vi "Suscribe To Audio Spectrum Notifier.vi"(8 "Error In":errorcluster, 11 "Display Manager In":refnum<class "Display Manager.lvclass">) -> (0 "Error Out":errorcluster, 3 "Display Manager Out":refnum<class "Display Manager.lvclass">)   [LabVIEW 2019, in "Display Manager.lvclass"]
uses:
  Display Manager.lvclass
  Accessors/Audio Spectrum Notifier/Set Audio Spectrum Notifier.vi
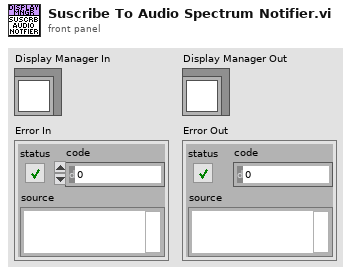
[diagram p1: front panel]
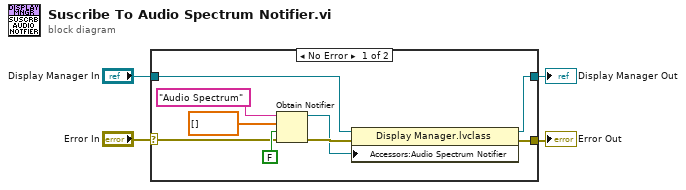
[diagram p0: block diagram]
diagram:
  n1 = case shown="No Error" "Error In" {
    selector: "Error In" -> [w7 w14]
    tunnel: [w13 w14] -> w4
    tunnel: [w12 w15] -> w3
    tunnel: "Display Manager In" -> [w9 w15]
    frame No Error {
      n2 = Obtain Notifier(name (unnamed)="Audio Spectrum", notification data type=dbl[] [], create if not found? (T)=FALSE, error in (no error)=w7) -> (notifier out=w10:refnum<notifier>, error out=w11:errorcluster)  [unwired: 1 out]
      n3 = property class="Display Manager.lvclass"(reference=w9, error in=w11, "Accessors:Audio Spectrum Notifier"=w10) -> (reference out=w12:refnum<class "Display Manager.lvclass">, error out=w13:errorcluster)
    }
    frame Error {
    }
  }
  "Error Out" <- w4
  "Display Manager Out" <- w3
